vi "PrintToPDF.vi"(0 "reference in":refnum<class "DP_WebView.lvclass">, 2 "PDF File path":path, 5 "Error In":errorcluster) -> (14 "reference out":refnum<class "DP_WebView.lvclass">, 15 "Result":bool, 16 "Status":i32(ring) items=["Created", "WaitingForActivation", "WaitingToRun", "Running", "WaitingForChildrenToComplete", "RanToCompletion", "Canceled", "Faulted"], 19 "Error Out":errorcluster)   [LabVIEW 2020, in "DP_WebView.lvclass"]
doc: "Get HTML comtent"
uses:
  DP_WebView.lvclass
  C:/Projects/DependencyViewer/DependencyViewer/DP_WebView_class/data/Microsoft.Web.WebView2.Core.dll
  data/Microsoft.Web.WebView2.Core.dll
  ctrls/ErrorCode.ctl
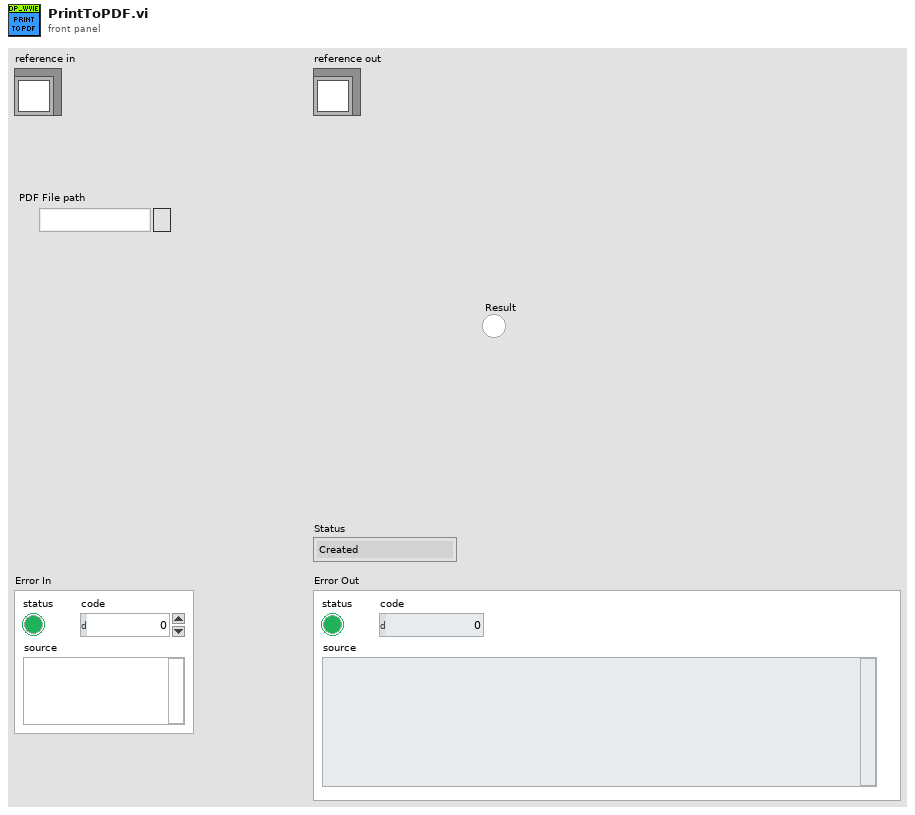
[diagram p1: front panel]
types:
  T1 = typedef "DP_WebView.lvclass/ErrorCode.ctl" = enum16{"Runtime engine is not installed or incompatible", "User Data Folder cannot be set", "Others", "JavaScript call failed", "PDF Printing Issue"}
  T2 = typedef "DP_WebView.lvclass/ObjectAttributes.ctl" = cluster{"WebView Container":refnum<k24>, "CoreWebViewRef":refnum<k24>, "Status":i32, "Status Message":string, "User Data Folder":path, "BrowserProcessId":u32}
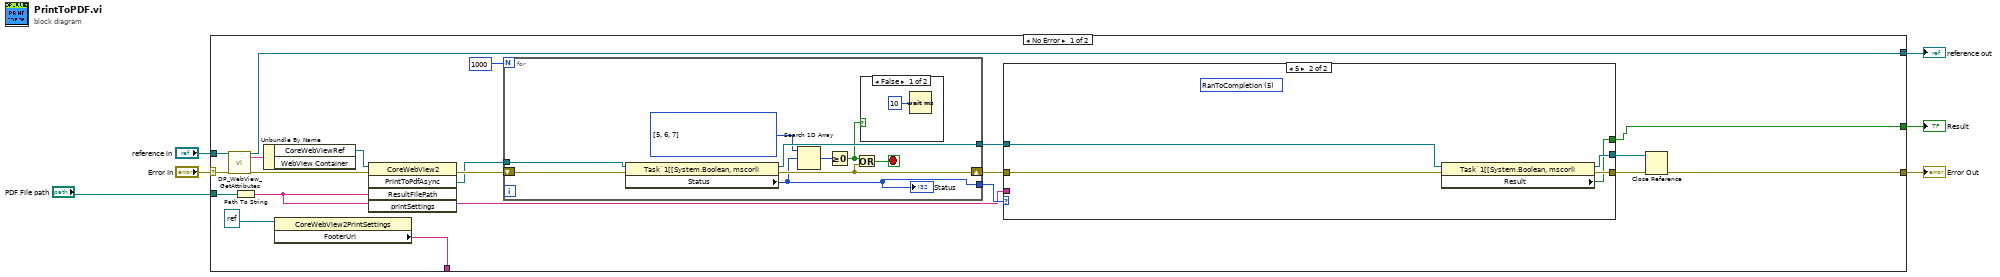
[diagram p0: block diagram]
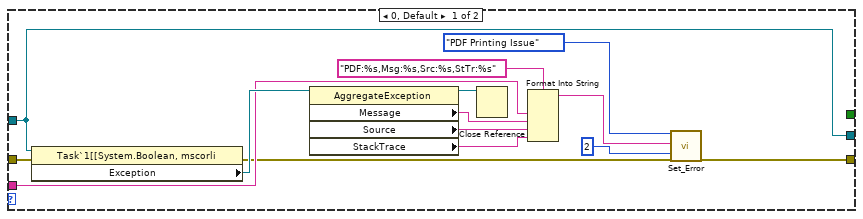
[diagram p2: hidden frame]
diagram:
  n1 = case shown="No Error" "Error In" {
    selector: "Error In" -> [w26 w57]
    tunnel: [w15 w57] -> w5
    tunnel: [w23 w56] -> w3
    tunnel: "reference in" -> [w24 w56]
    tunnel: [w7 _] -> w2
    tunnel: "PDF File path" -> [w11 _]
    tunnel: [w8 _] -> _
    frame No Error {
      n2 = call "DP_WebView_GetAttributes.vi"("reference in"=w24, "error in (no error)"=w26) -> ("reference out"=w23:refnum<class "DP_WebView.lvclass">, "Data"=w25:T2, "error out"=w22:errorcluster)  [unwired: 14 in, 1 out]
      n3 = Path To String(path=w11) -> (string=w10:string)
      n4 = Unbundle By Name(w25) -> ("CoreWebViewRef"=w13:refnum<k24>)  [unwired: 1 out]
      n5 = property class="CoreWebView2PrintSettings"(reference=refnum<k24> refnum ("printSettings")) -> ("FooterUri"=w8:string)  [unwired: 1 in, 2 out]
      n6 = invoke class="CoreWebView2" method="PrintToPdfAsync"(reference=w13, error in=w22, "ResultFilePath"=w10) -> (error out=w21:errorcluster, "PrintToPdfAsync"=w14:refnum<k24>)  [unwired: 2 in, 3 out]
      n7 = for {
        N: 1000 -> [_]
        tunnel: w14 -> [w54]
        shift-right: [w48] -> w18
        shift-left: w21 -> [w53]
        tunnel: [w52] -> w19
        tunnel: [w46] -> w12
        stop <- w47 stop-if-true
        w51 = i32[] [5, 6, 7] items=["Created", "WaitingForActivation", "WaitingToRun", "Running", "WaitingForChildrenToComplete", "RanToCompletion", "Canceled", "Faulted"] ("Status")
        n8 = property class="Task`1[[System.Boolean, mscorli"(reference=w54, error in=w53) -> (reference out=w52:refnum<k24>, error out=w48:errorcluster, "Status"=w46:i32)
        "Status" <- w46
        n9 = Search 1D Array(1D array=w51, element=w46) -> (index of element=w50:i32)  [unwired: 1 in]
        n10 = Greater Or Equal To 0?(x=w50) -> (x >= 0?=w49:bool)
        n11 = Or(x=w49, y=w48) -> (x .or. y?=w47:bool)
        n12 = case shown="False" w49 {
          frame False {
            n13 = Wait (ms)(milliseconds to wait=u32 10) -> ()  [unwired: 1 out]
          }
          frame True {
          }
        }
      }
      n14 = case shown="5" w12 {
        tunnel: w19 -> [w37 w45]
        tunnel: w18 -> [w36 w44]
        tunnel: [w37 w43] -> w17
        tunnel: [w40 w42] -> w16
        tunnel: [_ w41] -> w7
        tunnel: w10 -> [w33 _]
        frame 0, Default {
          n15 = property class="Task`1[[System.Boolean, mscorli"(reference=w37, error in=w36) -> (error out=w28:errorcluster, "Exception"=w35:refnum<k24>)  [unwired: 1 out]
          n16 = property class="AggregateException"(reference=w35) -> (reference out=w27:refnum<k24>, "Message"=w32:string, "Source"=w31:string, "StackTrace"=w30:string)  [unwired: 1 in, 1 out]
          n17 = Close Reference(reference=w27) -> ()  [unwired: 1 in, 1 out]
          n18 = Format Into String(format string="PDF:%s,Msg:%s,Src:%s,StTr:%s", w33, w32, w31, w30) -> (resulting string=w29:string)  [unwired: 2 in, 1 out]
          n19 = call "Set_Error.vi"("CustomErrors"=ErrorCode."PDF Printing Issue", "Description"=w29, "Error SubVI Level(1)"=2, "error in (no error)"=w28) -> ("error out"=w40:errorcluster)  [unwired: 15 in]
        }
        frame 5 {
          (unwired) 5 items=["Created", "WaitingForActivation", "WaitingToRun", "Running", "WaitingForChildrenToComplete", "RanToCompletion", "Canceled", "Faulted"] ("Status")
          n20 = property class="Task`1[[System.Boolean, mscorli"(reference=w45, error in=w44) -> (reference out=w43:refnum<k24>, error out=w42:errorcluster, "Result"=w41:bool)
        }
      }
      n21 = Close Reference(reference=w17, error in (no error)=w16) -> (error out=w15:errorcluster)
    }
    frame Error {
    }
  }
  "Error Out" <- w5
  "reference out" <- w3
  "Result" <- w2
